vi "Get Alternative Double Value.vi"(2 "Value":dbl, 3 "Min":dbl, 4 "Max":dbl) -> (0 "Alternative Value":dbl)   [LabVIEW 2020, in "Test.Camera.lvclass"]
uses:
  Test.Camera.lvclass
  Test.Camera.lvclass/Test.Camera.ctl
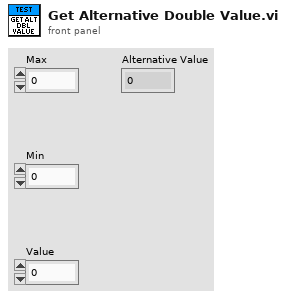
[diagram p1: front panel]
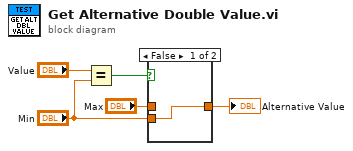
[diagram p0: block diagram]
diagram:
  n1 = Equal?(x="Value", y="Min") -> (x = y?=w4:bool)
  n2 = case shown="False" w4 {
    tunnel: [w6 w7] -> w2
    tunnel: "Max" -> [_ w7]
    tunnel: "Min" -> [w6 _]
    frame False {
    }
    frame True {
    }
  }
  "Alternative Value" <- w2
